vi "Fault Info VFD.vi"(8 "error In":errorcluster) -> (0 "error out":errorcluster, 2 "Faults":string[](array[string]), 3 "Fault":bool)   [LabVIEW 2026, in "VFD Library.lvlib"]
uses:
  VFD Library.lvlib
  Private/State Selection FGV.ctl
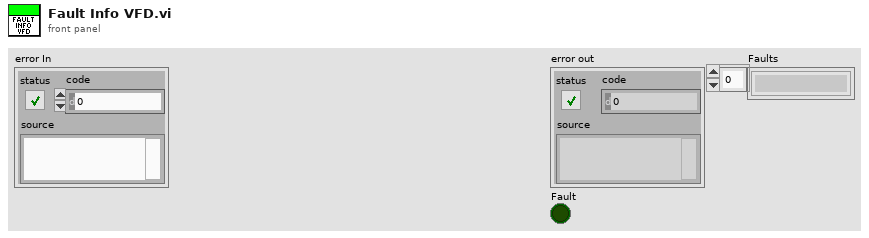
[diagram p1: front panel]
types:
  T1 = typedef "State Selection FGV.ctl" = enum16{"Initilize", "Write Reg", "Write Multiple Reg", "Read Reg", "Write Coil", "Read Coil", "Reset", "Close"}
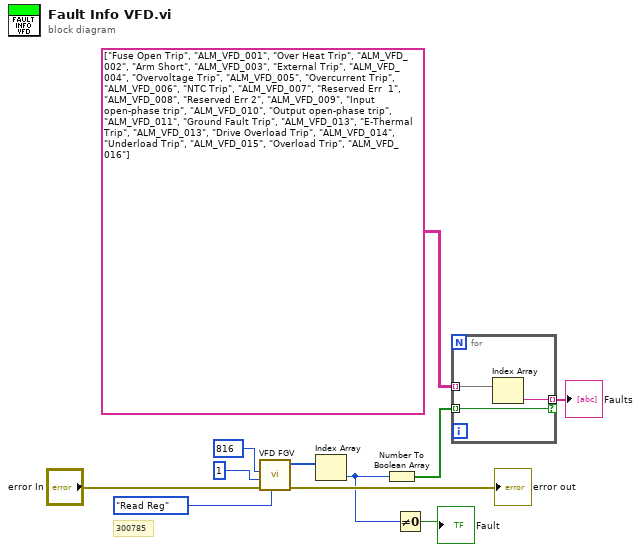
[diagram p0: block diagram]
diagram:
  # "300785"
  n1 = call "VFD FGV.vi"("State"=State_Selection_FGV."Read Reg", "error In"="error In", "value"=u16 1, "address"=u16 816) -> ("error out"=→"error out":errorcluster, "Registers"=w6:u16[])  [unwired: 5 in, 1 out]
  n2 = Index Array(array=w6) -> (element=w2:u16)  [unwired: 1 in]
  n3 = Number To Boolean Array(number=w2) -> (Boolean array=w5:bool[])
  n4 = Not Equal To 0?(x=w2) -> (x != 0?=→"Fault":bool)
  n5 = for {
    tunnel: w5 -> [w12] mode=indexing
    tunnel: string[][] [["Fuse Open Trip", "ALM_VFD_001"], ["Over Heat Trip", "ALM_VFD_002"], ["Arm Short", "ALM_VFD_003"], ["External Trip", "ALM_VFD_004"], ["Overvoltage Trip", "ALM_VFD_005"], ["Overcurrent Trip", "ALM_VFD_006"], ["NTC Trip", "ALM_VFD_007"], ["Reserved Err  1", "ALM_VFD_008"], ["Reserved Err 2", "ALM_VFD_009"], ["Input open-phase trip", "ALM_VFD_010"], ["Output open-phase trip", "ALM_VFD_011"], ["Ground Fault Trip", "ALM_VFD_013"], ["E-Thermal Trip", "ALM_VFD_013"], ["Drive Overload Trip", "ALM_VFD_014"], ["Underload Trip", "ALM_VFD_015"], ["Overload Trip", "ALM_VFD_016"]] -> [w14] mode=indexing
    tunnel: [w13] -> w3 mode=indexing if=w12
    n6 = Index Array(array=w14) -> (element=w13:string)  [unwired: 1 in]
  }
  "Faults" <- w3
